vi "week5_array_cluster_LV18.vi"() -> ()   [LabVIEW 2018]
panel:
  in  "Number to insert into array":dbl
  in  "Array element location to insert":dbl=-1.0
  out "Sub-array":dbl[](array[numeric])
  in  "Array subset length":dbl
  in  "Array subset start no.":dbl
  out "Array max":dbl
  out "Array min":dbl
  in  "Number to replace into array":dbl
  in  "Array element no. to replace":dbl=-1.0
  in  "stop":bool
  out "Array element":dbl
  in  "Array element no.":sgl
  out "Array mean":dbl
  out "Cluster":T1
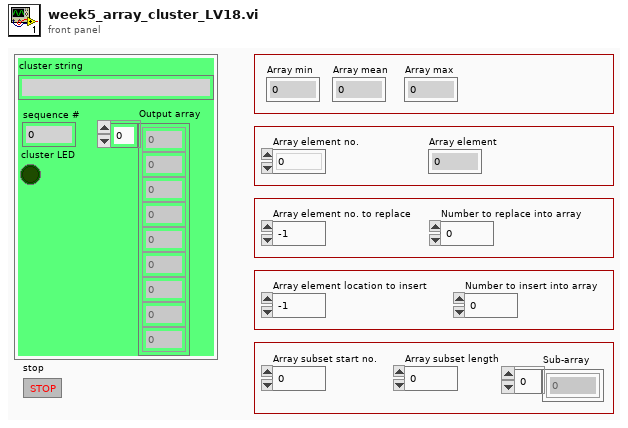
[diagram p1: front panel]
types:
  T1 = cluster{"cluster string":string, "sequence #":dbl, "cluster LED":bool, "Output array":dbl[]}
  T2 = cluster{"cluster name":string, i32, "cluster bool":bool, i32[]}
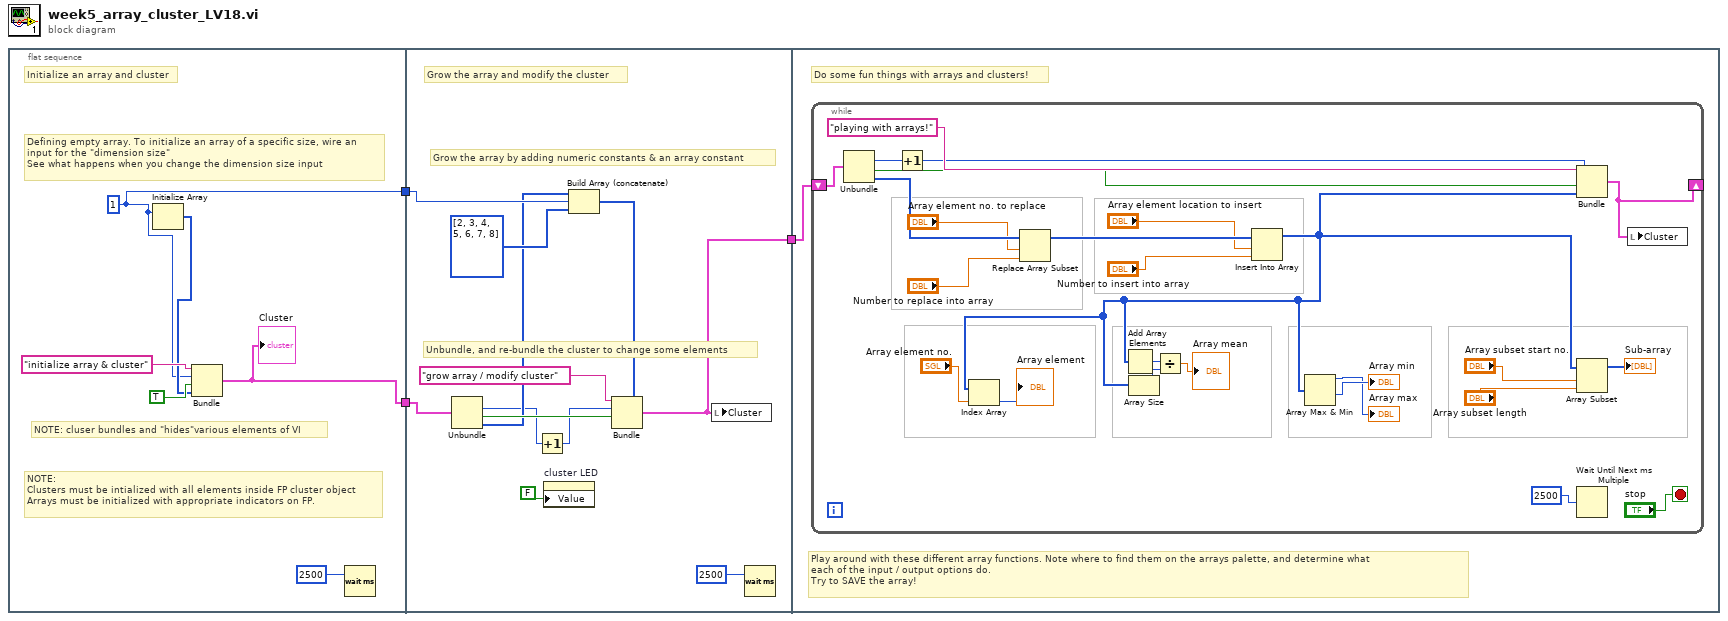
[diagram p0: block diagram]
diagram:
  n1 = flat-sequence {
    tunnel: [w5] -> w3
    tunnel: [w4] -> w2
    tunnel: w3 -> [w21]
    tunnel: w2 -> [w19]
    tunnel: [w12] -> w1
    tunnel: w1 -> [w22]
    frame #0 {
      w5 = 1
      # "NOTE:\nClusters must be intialized with all elements inside FP cluster object\nArrays must be initialized with appropriate indicators on FP."
      # "Defining empty array. To initialize an array of a specific size, wire an \ninput for the \"dimension size\"\nSee what happens when you change the dimension size input"
      # "NOTE: cluser bundles and \"hides\"various elements of VI"
      # "Initialize an array and cluster"
      n2 = Initialize Array(w5) -> (w7:i32[])  [unwired: 1 in]
      n3 = Bundle("cluster name"="initialize array & cluster", w5, "cluster bool"=TRUE, w7) -> (w4:T2)  [unwired: 1 in]
      "Cluster" <- w4
      n4 = Wait (ms)(milliseconds to wait=2500) -> ()  [unwired: 1 out]
    }
    frame #1 {
      # "Unbundle, and re-bundle the cluster to change some elements"
      # "Grow the array by adding numeric constants & an array constant"
      # "Grow the array and modify the cluster"
      n5 = Unbundle(w19) -> (w15:i32, "cluster bool"=w18:bool, w17:i32[])  [unwired: 1 out]
      n6 = Increment(x=w15) -> (x+1=w14:i32)
      n7 = property on="cluster LED" class="Bool (strict)"("Value"=FALSE) -> ()  [unwired: 2 in, 2 out]
      n8 = Build Array (concatenate)(w17, w21, i32[] [2, 3, 4, 5, 6, 7, 8]) -> (w16:i32[])
      n9 = Bundle("cluster name"="grow array / modify cluster", w14, "cluster bool"=w18, w16) -> (w12:T2)  [unwired: 1 in]
      n10 = local write "Cluster"(w12) -> ()
      n11 = Wait (ms)(milliseconds to wait=2500) -> ()  [unwired: 1 out]
    }
    frame #2 {
      # "Play around with these different array functions. Note where to find them on the arrays palette, and determine what \neach of the input / output options do.\nTry to SAVE the array!"
      # "Do some fun things with arrays and clusters!"
      n12 = while {
        shift-right: [w38] -> _
        shift-left: w22 -> [w37]
        stop <- "stop" stop-if-true
        n13 = Unbundle(w37) -> (w46:i32, "cluster bool"=w44:bool, w34:i32[])  [unwired: 1 out]
        n14 = Increment(x=w46) -> (x+1=w45:i32)
        n15 = Replace Array Subset "Replace Array Subset"(array=w34, new element="Number to replace into array", index="Array element no. to replace") -> (w26:i32[])
        n16 = Insert Into Array "Insert Into Array"(array=w26, index="Array element location to insert", new element="Number to insert into array") -> (w23:i32[])
        n17 = Index Array "Index Array"(array=w23, index="Array element no.") -> (element=→"Array element":i32)
        n18 = Add Array Elements(numeric array=w23) -> (sum=w43:i32)
        n19 = Array Size(array=w23) -> (size(s)=w42:i32)
        n20 = Divide(x=w43, y=w42) -> (x/y=→"Array mean":dbl)
        n21 = Array Max & Min(array=w23) -> (max value=→"Array max":i32, min value=→"Array min":i32)  [unwired: 2 out]
        n22 = Bundle("playing with arrays!", w45, "cluster bool"=w44, w23) -> (w38:cluster{string, i32, "cluster bool":bool, i32[]})  [unwired: 1 in]
        n23 = Array Subset "Array Subset"(array=w23, index="Array subset start no.", length="Array subset length") -> (→"Sub-array":i32[])
        n24 = Wait Until Next ms Multiple(millisecond multiple=2500) -> ()  [unwired: 1 out]
        n25 = local write "Cluster"(w38) -> ()
      }
    }
  }
